vi "MGI Topological Sort.vi"(8 "error in (no error)":errorcluster, 10 "Nodes":T1[](array[typedef])) -> (0 "error out":errorcluster, 2 "Sorted Pointers":i32[](array[numeric]))   [LabVIEW 2016]
doc: "Topologically Sorts a Directed Graph. Only graphs with no circular dependancies can be sorted.\n\nImplements Khan's Algorithm as described here: https://en.wikipedia.org/wiki/Topological_sorting\n\nCopyright: MGI 2016\nAuthor: Derek Trepanier"
uses:
  <userlib>/_MGI/1D Array/MGI Topological Node.ctl
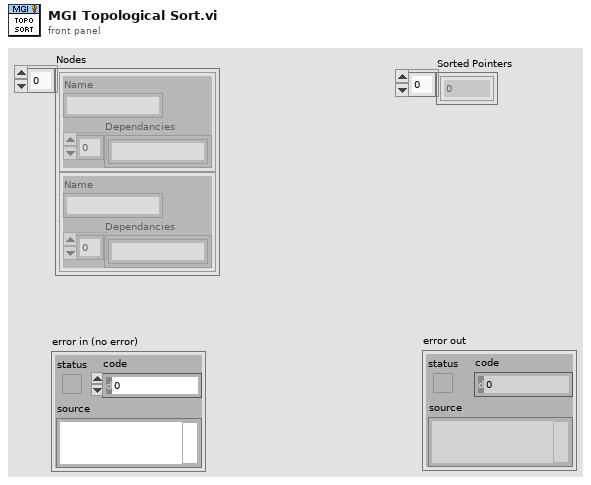
[diagram p1: front panel]
types:
  T1 = typedef "MGI Topological Node.ctl" = cluster{"Name":string, "Dependancies":string[]}
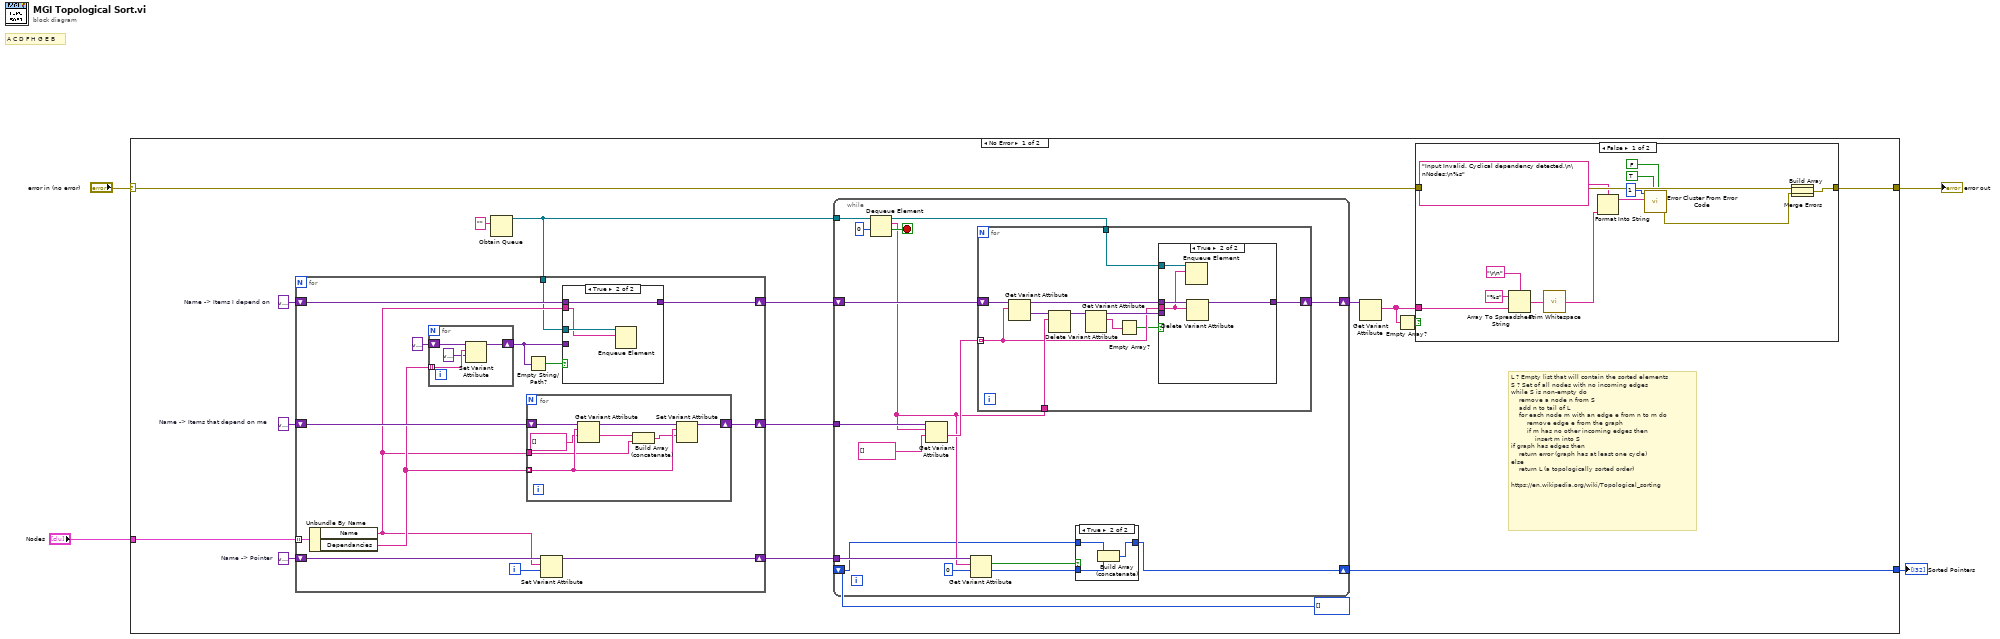
[diagram p0: block diagram]
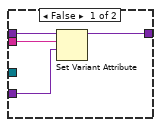
[diagram p3: hidden frame]
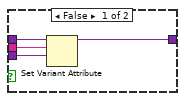
[diagram p5: hidden frame]
diagram:
  # "A C D F H G E B"
  n1 = case shown="No Error" "error in (no error)" {
    selector: "error in (no error)" -> [w11 w108]
    tunnel: "Nodes" -> [w7 _]
    tunnel: [w10 w108] -> w2
    tunnel: [w6 _] -> w1
    frame No Error {
      w15 = variant  # Name -> Pointer
      w17 = variant  # Name -> Items that depend on me
      w19 = variant  # Name -> Items I depend on
      # "L ? Empty list that will contain the sorted elements\nS ? Set of all nodes with no incoming edges\nwhile S is non-empty do\n    remove a node n from S\n    add n to tail of L\n    for each node m with an edge e from n to m do\n        remove edge e from the graph\n        if m has no other incoming edges then\n            insert m into S\nif graph has edges then\n    return error (graph has at least one cycle)\nelse \n    return L (a topologically sorted order)\n\nhttps://en.wikipedia.org/wiki/Topological_sorting"
      n2 = Obtain Queue(element data type="") -> (queue out=w13:refnum<queue>)  [unwired: 4 in, 2 out]
      n3 = for {
        tunnel: w7 -> [w49] mode=indexing
        tunnel: w13 -> [w36]
        shift-right: [w47] -> w18
        shift-left: w19 -> [w48]
        shift-right: [w45] -> w16
        shift-left: w17 -> [w46]
        shift-right: [w42] -> w14
        shift-left: w15 -> [w43]
        i -> [w40]
        n4 = Unbundle By Name(w49) -> ("Name"=w41:string, "Dependancies"=w44:string[])
        n5 = for {
          shift-right: [w60] -> w38
          shift-left: variant -> [w59]
          tunnel: w44 -> [w58] mode=indexing
          n6 = Set Variant Attribute(Variant=w59, name=w58, value=variant) -> (Variant out=w60:variant)  [unwired: 1 in, 2 out]
        }
        n7 = for {
          shift-right: [w61] -> w45
          shift-left: w46 -> [w68]
          tunnel: w44 -> [w66] mode=indexing
          tunnel: w41 -> [w63]
          n8 = Get Variant Attribute(Variant=w68, name=w66, default value (empty Variant)=string[] [] ("Dependancies")) -> (duplicate Variant=w67:variant, value=w65:string[])  [unwired: 1 in, 2 out]
          n9 = Build Array (concatenate)(w65, w63) -> (w64:string[])
          n10 = Set Variant Attribute(Variant=w67, name=w66, value=w64) -> (Variant out=w61:variant)  [unwired: 1 in, 2 out]
        }
        n11 = Empty String/Path?(string/path=w38) -> (empty?=w37:bool)
        n12 = Set Variant Attribute(Variant=w43, name=w41, value=w40) -> (Variant out=w42:variant)  [unwired: 1 in, 2 out]
        n13 = case shown="True" w37 {
          tunnel: w48 -> [w53 w56]
          tunnel: [w52 w56] -> w47
          tunnel: w41 -> [w51 w54]
          tunnel: w38 -> [w50 _]
          tunnel: w36 -> [_ w55]
          frame False {
            n14 = Set Variant Attribute(Variant=w53, name=w51, value=w50) -> (Variant out=w52:variant)  [unwired: 1 in, 2 out]
          }
          frame True {
            n15 = Enqueue Element(queue=w55, element=w54) -> ()  [unwired: 2 in, 3 out]
          }
        }
      }
      n16 = while {
        shift-right: [w79] -> w12
        shift-left: w18 -> [w83]
        tunnel: w16 -> [w82]
        tunnel: w14 -> [w76]
        tunnel: w13 -> [w71]
        shift-right: [w69] -> w6
        shift-left: i32[] [] ("Array") -> [w70]
        stop <- w77 stop-if-true
        n17 = Dequeue Element(queue=w71, timeout in ms (-1)=0) -> (queue out=w78:refnum<queue>, element=w75:string, timed out?=w77:bool)  [unwired: 1 in, 1 out]
        n18 = Get Variant Attribute(Variant=w82, name=w75, default value (empty Variant)=string[] [] ("Dependancies")) -> (value=w80:string[])  [unwired: 1 in, 3 out]
        n19 = Get Variant Attribute(Variant=w76, name=w75, default value (empty Variant)=0) -> (found=w72:bool, value=w73:i32)  [unwired: 1 in, 2 out]
        n20 = for {
          tunnel: w80 -> [w91] mode=indexing
          shift-right: [w96] -> w79
          shift-left: w83 -> [w99]
          tunnel: w75 -> [w95]
          tunnel: w78 -> [w89]
          n21 = Get Variant Attribute(Variant=w99, name=w91) -> (duplicate Variant=w98:variant, value=w97:variant)  [unwired: 2 in, 2 out]
          n22 = Delete Variant Attribute(6:w95, 7:w97) -> (3:w94:variant)  [unwired: 1 in, 2 out]
          n23 = Get Variant Attribute(Variant=w94) -> (duplicate Variant=w93:variant, names=w92:string[])  [unwired: 3 in, 2 out]
          n24 = Empty Array?(array=w92) -> (empty?=w90:bool)
          n25 = case shown="True" w90 {
            tunnel: w98 -> [w103 w107]
            tunnel: [w102 w106] -> w96
            tunnel: w93 -> [w101 _]
            tunnel: w91 -> [w100 w104]
            tunnel: w89 -> [_ w105]
            frame False {
              n26 = Set Variant Attribute(Variant=w103, name=w100, value=w101) -> (Variant out=w102:variant)  [unwired: 1 in, 2 out]
            }
            frame True {
              n27 = Enqueue Element(queue=w105, element=w104) -> ()  [unwired: 2 in, 3 out]
              n28 = Delete Variant Attribute(6:w104, 7:w107) -> (3:w106:variant)  [unwired: 1 in, 2 out]
            }
          }
        }
        n29 = case shown="True" w72 {
          tunnel: w70 -> [w85 w87]
          tunnel: w73 -> [_ w86]
          tunnel: [w85 w88] -> w69
          frame False {
          }
          frame True {
            n30 = Build Array (concatenate)(w87, w86) -> (w88:i32[])
          }
        }
      }
      n31 = Get Variant Attribute(Variant=w12) -> (names=w8:string[])  [unwired: 3 in, 3 out]
      n32 = Empty Array?(array=w8) -> (empty?=w9:bool)
      n33 = case shown="False" w9 {
        tunnel: w11 -> [w34 w35]
        tunnel: [w33 w35] -> w10
        tunnel: w8 -> [w31 _]
        frame False {
          n34 = Array To Spreadsheet String(delimiter (Tab)="\r\n", array=w31, 3:"%s" ("format string")) -> (spreadsheet string=w28:string)
          n35 = call <vilib>:"Trim Whitespace.vi"("string"=w28) -> ("trimmed string"=w27:string)  [unwired: 1 in]
          n36 = Format Into String(format string="Input Invalid. Cyclical dependency detected.\n\nNodes:\n%s", w27) -> (resulting string=w24:string)  [unwired: 2 in, 1 out]
          n37 = call <vilib>:"Error Cluster From Error Code.vi"("is warning? (False)"=FALSE, "show call chain? (False)"=TRUE, "error message (\"\")"=w24, "error code (0)"=1) -> ("error out"=w32:errorcluster)  [unwired: 5 in]
          n38 = Build Array(w34, w32) -> (w21:errorcluster[])
          n39 = Merge Errors(w21) -> (w33:errorcluster)
        }
        frame True {
        }
      }
    }
    frame Error {
    }
  }
  "error out" <- w2
  "Sorted Pointers" <- w1
